vi "preparetiffs.vi"(2 "filename prefix":string, 3 "data dir":path=path "C:/Users/Labmember/Desktop/Data/temp" caption="data dir.", 4 "timestamp":timestamp) -> (1 "full-filename":string="20140304-163843-")   [LabVIEW 2015]
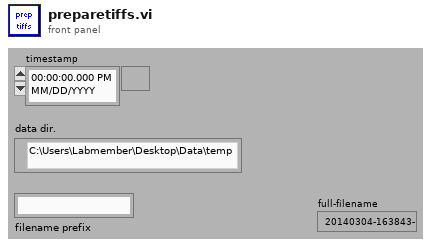
[diagram p1: front panel]
types:
  T1 = typedef "LVRectTypeDef.ctl" = cluster{"Left":i16, "Top":i16, "Right":i16, "Bottom":i16}
  T2 = cluster{"Xpixels":i32, "Vxminref":dbl, "Vxmaxref":dbl, "P":dbl, "Ypixels":i32, "Vyminref":dbl, "Vymaxref":dbl, "srate":sgl, "sAOxy":i32, "timeout":dbl, "type":string, "date":string, "time":string, "Colormap":u16, "Drawing Mode":u16, "Scanning Mode":u16, "square pixels":bool, "square matrix":bool, "Xpixels Img":i32, "Vx-min Img":dbl, "VX-max Img":dbl, "Ypixels Img":i32, "Vy-min Img":dbl, "Vy-max Img ":dbl, "Angle Img":dbl, "autoshutter":bool, "finite":bool, "cont":bool, "wavdet":bool, "measpoints":i32, "avpp":i32, "bufferAO":i32, "bufferAI":i32, "starttick":u32, "waveform":path, "Vx-ref":dbl, "Vy-ref":dbl, "refreshrate":dbl, "refreshbuffer":i32, "tt_cycles":i32, "motorref":refnum<k7>, "mirrorswitch":refnum<k7>, "sample mode":i32, "maxbufferAI":i32, "srateAODO":sgl, "bin":sgl, "Pel":sgl, "Angle draw":dbl, "srate Img":sgl, "ROIimg_plotbounds":T1, "auto OD":bool, "ODfilt":u16, "aAI":i32[], "aCI":i32[], "aAO":u32[], "aDO":u32[], "refwfsize":dbl, "Lifetime":bool, "Vz-Img":dbl, "Vz-ref":dbl, "Vz-reset":dbl, "AIoverride":bool}
  T3 = typedef "XYZStage.lvlib/XYZStage Configuration.ctl" = cluster{"VISA resource name":refnum<visa-resource-name>, "Timeout (3sec)":u32}
  T4 = cluster{"StageS":i32, "StageL":i32, "currmeas data dir":path, "image OD":u16, "contour OD":u16, "point OD":u16, "AOlines":tag[], "AIlines":tag[], "CI lines":tag[], "DO lines":tag[], "AO names":string[], "CI names":string[], "AI names":string[], "DO names":string[], "CIextensions":string[], "AIextensions":string[], "Voltage to Ygalvo":i32, "Voltage to Xgalvo":i32, "Voltage to patch":i32, "640 shutter":i32, "2P shutter":i32, "LT timestamp":u32, "Vp":i32, "Ip":i32, "camera trigger":i32, "master data dir":path, "voltage to Zpos":i32, "Vto2P":i32, "640 AO":i32, "488 AO":i32, "532 AO":i32, "640TTL":u32, "488TTL":u32, "532TTL":u32, "Device 1 sampleclock out":tag, "Device 1 Starttrigger out":tag, "Device 2 sampleclock in":tag, "Device 2 StartTrigger in ":tag, "2PODTTL":u32, "488 shutter":u32, "LCVR red":u32, "LCVR blue":u32, "Sutter Stage Config":T3}
  T5 = cluster{"filetif":refnum<file>[], "E_filetif":errorcluster[]}
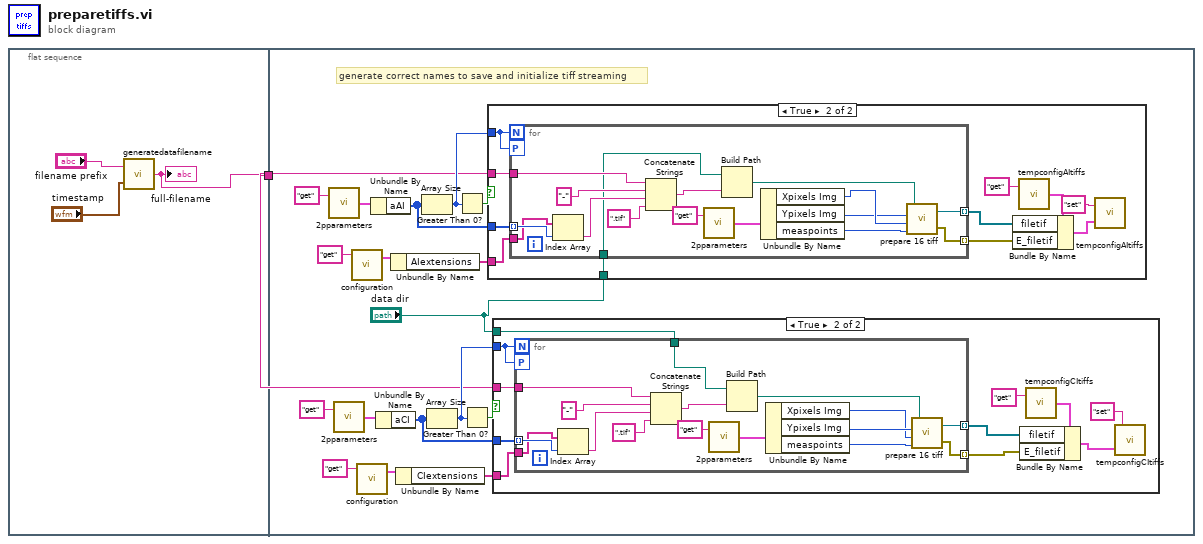
[diagram p0: block diagram]
diagram:
  n1 = flat-sequence {
    tunnel: [w2] -> w1
    tunnel: w1 -> [w6]
    frame #0 {
      n2 = call "generatedatafilename.vi"("timestamp"="timestamp", "filename prefix in"="filename prefix") -> ("full-filename"=w2:string)
      "full-filename" <- w2
    }
    frame #1 {
      # "generate correct names to save and initialize tiff streaming"
      n3 = call "2pparameters.vi"("command"="get") -> ("params out"=w22:T2)  [unwired: 1 in]
      n4 = call "2pparameters.vi"("command"="get") -> ("params out"=w7:T2)  [unwired: 1 in]
      n5 = call "configuration.vi"("command"="get") -> ("config out"=w20:T4)  [unwired: 2 in, 1 out]
      n6 = call "configuration.vi"("command"="get") -> ("config out"=w9:T4)  [unwired: 2 in, 1 out]
      n7 = Unbundle By Name(w22) -> ("aAI"=w16:i32[])
      n8 = Unbundle By Name(w7) -> ("aCI"=w13:i32[])
      n9 = Unbundle By Name(w20) -> ("AIextensions"=w15:string[])
      n10 = Unbundle By Name(w9) -> ("CIextensions"=w14:string[])
      n11 = Array Size(array=w16) -> (size(s)=w17:i32)
      n12 = Array Size(array=w13) -> (size(s)=w12:i32)
      n13 = Greater Than 0?(x=w17) -> (x > 0?=w18:bool)
      n14 = Greater Than 0?(x=w12) -> (x > 0?=w11:bool)
      n15 = case shown="True" w18 {
        tunnel: w17 -> [_ w60]
        tunnel: w16 -> [_ w59]
        tunnel: w15 -> [_ w58]
        tunnel: w6 -> [_ w51]
        tunnel: "data dir" -> [_ w50]
        frame False {
        }
        frame True {
          n16 = for {
            N: w60 -> [_]
            workers-P: w60 -> [_]
            tunnel: w59 -> [w70] mode=indexing
            tunnel: w58 -> [w69]
            tunnel: [w66] -> w53 mode=indexing
            tunnel: [w65] -> w52 mode=indexing
            tunnel: w51 -> [w64]
            tunnel: w50 -> [w63]
            n17 = Index Array(array=w69, index=w70) -> (element=w67:string)
            n18 = Concatenate Strings(w64, "-" ("string"), w67, ".tif" ("string")) -> (w75:string)
            n19 = call "2pparameters.vi"("command"="get") -> ("params out"=w72:T2)  [unwired: 1 in]
            n20 = Build Path(base path=w63, name or relative path=w75) -> (appended path=w74:path)
            n21 = Unbundle By Name(w72) -> ("Xpixels Img"=w62:i32, "Ypixels Img"=w61:i32, "measpoints"=w71:i32)
            n22 = call "prepare 16 tiff.vi"("z"=w71, "y"=w62, "x"=w61, "file path"=w74) -> ("error out"=w65:errorcluster, "refnum tif"=w66:refnum<file>)
          }
          n23 = call "tempconfigAItiffs.vi"("command"="get") -> ("Temp Config out"=w56:T5)  [unwired: 1 in]
          n24 = Bundle By Name(cluster=w56, "filetif"=w53, "E_filetif"=w52) -> (w57:T5)
          n25 = call "tempconfigAItiffs.vi"("Temp Config in"=w57, "command"="set") -> ()  [unwired: 1 out]
        }
      }
      n26 = case shown="True" w11 {
        tunnel: w12 -> [_ w33]
        tunnel: w13 -> [_ w32]
        tunnel: w14 -> [_ w31]
        tunnel: w6 -> [_ w28]
        tunnel: "data dir" -> [_ w23]
        frame False {
        }
        frame True {
          n27 = for {
            N: w33 -> [_]
            workers-P: w33 -> [_]
            tunnel: w32 -> [w43] mode=indexing
            tunnel: w31 -> [w42]
            tunnel: [w39] -> w30 mode=indexing
            tunnel: [w38] -> w29 mode=indexing
            tunnel: w28 -> [w37]
            tunnel: w23 -> [w36]
            n28 = Index Array(array=w42, index=w43) -> (element=w40:string)
            n29 = Concatenate Strings(w37, "-" ("string"), w40, ".tif" ("string")) -> (w48:string)
            n30 = call "2pparameters.vi"("command"="get") -> ("params out"=w45:T2)  [unwired: 1 in]
            n31 = Build Path(base path=w36, name or relative path=w48) -> (appended path=w47:path)
            n32 = Unbundle By Name(w45) -> ("Xpixels Img"=w34:i32, "Ypixels Img"=w35:i32, "measpoints"=w44:i32)
            n33 = call "prepare 16 tiff.vi"("z"=w44, "y"=w34, "x"=w35, "file path"=w47) -> ("error out"=w38:errorcluster, "refnum tif"=w39:refnum<file>)
          }
          n34 = call "tempconfigCItiffs.vi"("command"="get") -> ("Temp Config out"=w26:T5)  [unwired: 1 in]
          n35 = Bundle By Name(cluster=w26, "filetif"=w30, "E_filetif"=w29) -> (w25:T5)
          n36 = call "tempconfigCItiffs.vi"("Temp Config in"=w25, "command"="set") -> ()  [unwired: 1 out]
        }
      }
    }
  }
